vi "Serial Comm.vi"(4 "Timeout (ms)":u32=1000, 6 "Expected Bytes":u32=100, 7 "Query?":bool, 8 "error in (no error)":errorcluster, 9 "End of Response":string="\r\n", 10 "Command":string, 11 "VISA resource name in":refnum<visa-resource-name>) -> (0 "error out":errorcluster, 2 "Response":string, 3 "VISA resource name out":refnum<visa-resource-name>)   [LabVIEW 2015]
uses:
  Utilities.lvlib
panel:
  out "Elapsed Time (ms)":u32
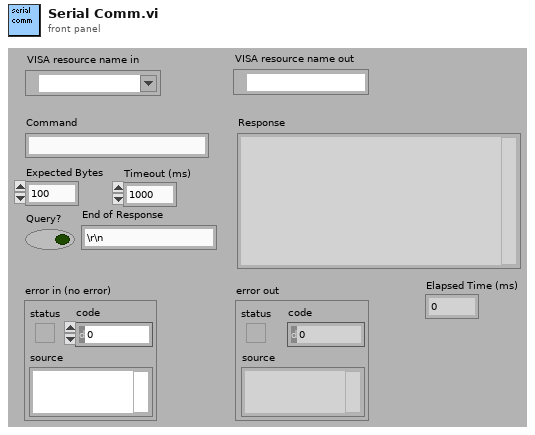
[diagram p1: front panel]
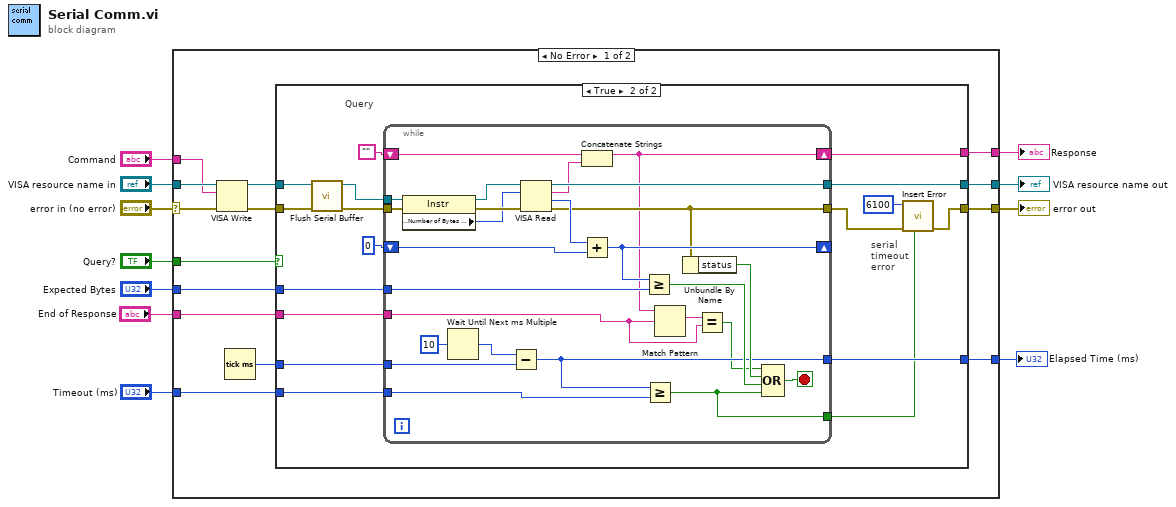
[diagram p0: block diagram]
diagram:
  n1 = case shown="No Error" "error in (no error)" {
    selector: "error in (no error)" -> [w25 w72]
    tunnel: [w24 w72] -> w10
    tunnel: "VISA resource name in" -> [w22 w71]
    tunnel: [w20 w71] -> w8
    tunnel: "Command" -> [w19 _]
    tunnel: "Query?" -> [w18 _]
    tunnel: "Expected Bytes" -> [w17 _]
    tunnel: [w16 _] -> w4
    tunnel: "Timeout (ms)" -> [w14 _]
    tunnel: [w13 _] -> w2
    tunnel: "End of Response" -> [w12 _]
    frame No Error {
      n2 = VISA Write(VISA resource name=w22, write buffer=w19, error in (no error)=w25) -> (VISA resource name out=w21:refnum<visa-resource-name>, error out=w23:errorcluster)  [unwired: 1 out]
      n3 = Tick Count (ms)() -> (millisecond timer value=w15:u32)
      n4 = case shown="True" w18 {
        tunnel: [w26 w36] -> w24
        tunnel: w23 -> [w26 w30]
        tunnel: w21 -> [w27 w32]
        tunnel: [w27 w44] -> w20
        tunnel: w17 -> [_ w42]
        tunnel: [_ w41] -> w16
        tunnel: w15 -> [_ w39]
        tunnel: w14 -> [_ w38]
        tunnel: [_ w37] -> w13
        tunnel: w12 -> [_ w28]
        frame False {
          # "Command"
        }
        frame True {
          # "serial \ntimeout\nerror"
          # "Query"
          n5 = call "Flush Serial Buffer.vi"("error in (no error)"=w30, "VISA resource name in"=w32) -> ("error out"=w29:errorcluster, "VISA resource name out"=w31:refnum<visa-resource-name>)  [unwired: 8 in]
          n6 = while {
            tunnel: [w56] -> w35
            tunnel: w29 -> [w70]
            tunnel: w31 -> [w68]
            tunnel: [w66] -> w44
            shift-right: [w48] -> w41
            shift-left: "" -> [w63]
            tunnel: w42 -> [w58]
            shift-right: [w59] -> _
            shift-left: u32 0 -> [w60]
            tunnel: w39 -> [w52]
            tunnel: w38 -> [w51]
            tunnel: [w50] -> w37
            tunnel: [w49] -> w34
            tunnel: w28 -> [w46]
            stop <- w62 stop-if-true
            n7 = property class="Instr"(reference=w68, error in=w70) -> (reference out=w67:refnum<visa-resource-name>, error out=w69:errorcluster, "Serial Settings:Number of Bytes at Serial Port"=w65:u32)
            n8 = Wait Until Next ms Multiple(millisecond multiple=u32 10) -> (millisecond timer value=w53:u32)
            n9 = Subtract(x=w53, y=w52) -> (x-y=w50:u32)
            n10 = VISA Read(VISA resource name=w67, byte count=w65, error in (no error)=w69) -> (VISA resource name out=w66:refnum<visa-resource-name>, read buffer=w64:string, return count=w61:u32, error out=w56:errorcluster)
            n11 = Concatenate Strings(w63, w64) -> (w48:string)
            n12 = Add(x=w61, y=w60) -> (x+y=w59:u32)
            n13 = Greater Or Equal?(x=w59, y=w58) -> (x >= y?=w57:bool)
            n14 = Greater Or Equal?(x=w50, y=w51) -> (x >= y?=w49:bool)
            n15 = Match Pattern(string=w48, regular expression=w46) -> (match substring=w47:string)  [unwired: 1 in, 3 out]
            n16 = Unbundle By Name(w56) -> ("status"=w55:bool)
            n17 = Equal?(x=w47, y=w46) -> (x = y?=w45:bool)
            n18 = Compound Arithmetic op=OR(w45, w55, w57, w49) -> (w62:bool)
          }
          n19 = call "Insert Error.vi"("[error code] (0)"=6100, "error in (no error)"=w35, "error?"=w34) -> ("error out"=w36:errorcluster)  [unwired: 7 in]
        }
      }
    }
    frame Error {
    }
  }
  "error out" <- w10
  "VISA resource name out" <- w8
  "Response" <- w4
  "Elapsed Time (ms)" <- w2
